vi "sig_test.vi"(2 "index (row)":i32) -> (0 "element":dbl format="%#_16f")   [LabVIEW 2010]
panel:
  out "array":dbl[][](array[numeric]) format="%_16f"
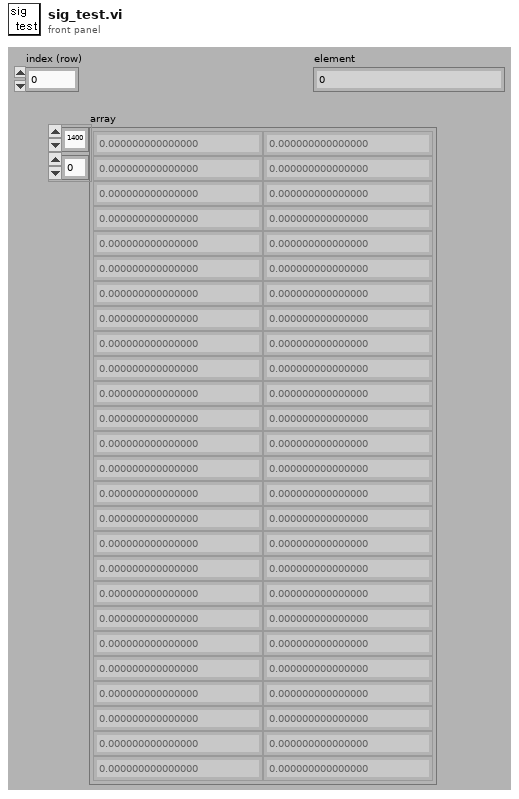
[diagram p1: front panel]
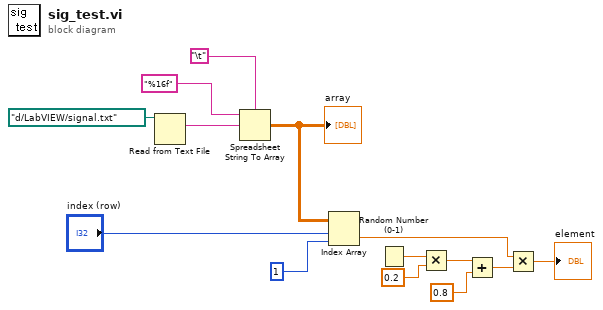
[diagram p0: block diagram]
diagram:
  n1 = Read from Text File(file (use dialog)=path "d:/LabVIEW/signal.txt") -> (text=w13:string)  [unwired: 3 in, 3 out]
  n2 = Spreadsheet String To Array(delimiter (Tab)="\t", format string="%16f", spreadsheet string=w13) -> (array=w10:dbl[][])  [unwired: 1 in]
  "array" <- w10
  n3 = Index Array(array=w10, index (row)="index (row)", index (col)=1 ("disabled index (col)")) -> (element=w2:dbl)
  n4 = Random Number (0-1)() -> (number: 0 to 1=w7:dbl)
  n5 = Multiply(x=w7, y=0.2) -> (x*y=w5:dbl)
  n6 = Add(x=w5, y=0.8) -> (x+y=w3:dbl)
  n7 = Multiply(x=w2, y=w3) -> (x*y=→"element":dbl)
